vi "PPMS_CREA_SECUENCIA.vi"(8 "error in (no error)":errorcluster) -> (0 "error out":errorcluster, 1 "Total":string[](array[string]), 2 "Pasos":i32, 3 "Secuencia":string[](array[string]))   [LabVIEW 2017]
uses:
  <vilib>/Utility/file.llb/Read Delimited Spreadsheet (string).vi
panel:
  out "idxScanVi":i16
  out "idxScanVf":i16
  out "Scan V":bool
  out "subArray2D":string[][](array[string])
  out "Seq scans":string[](array[string])
  out "Seq final":string[](array[string])
  out "Seq inicial":string[](array[string])
  out "idxScanTi":i16
  out "idxScanFi":i16
  out "idxScanFf":i16
  out "idxScanTf":i16
  out "Array2D":string[][](array[string])
  out "Scan T":bool
  out "Scan F":bool
  in  "Salir":bool
  in  "Borra linea":bool
  in  "Grabar":bool
  in  "Cargar":bool
  out "SequenceFile":path
  in  "Command line (double click)":i32(listbox) caption="Válvulas"
  in  "Secuencia":i32(listbox)=-1
  # "Septiembre 2019 V1.2  a-sslcdms"
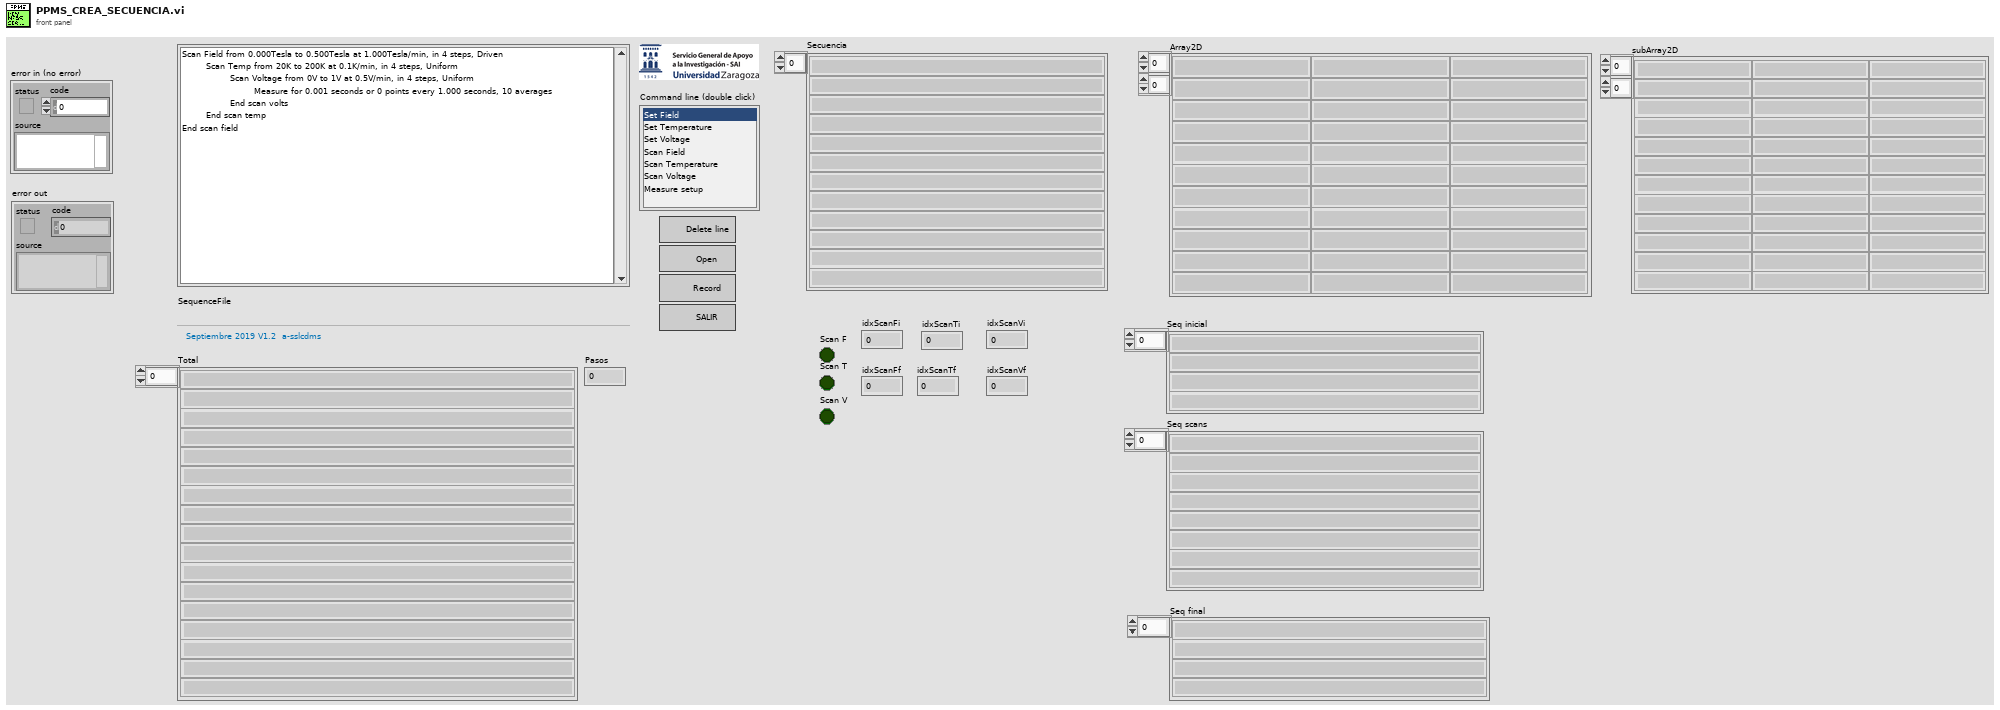
[diagram p1: front panel]
types:
  T1 = enum16{"open", "open or create", "create or replace", "create", "open (read only)"}
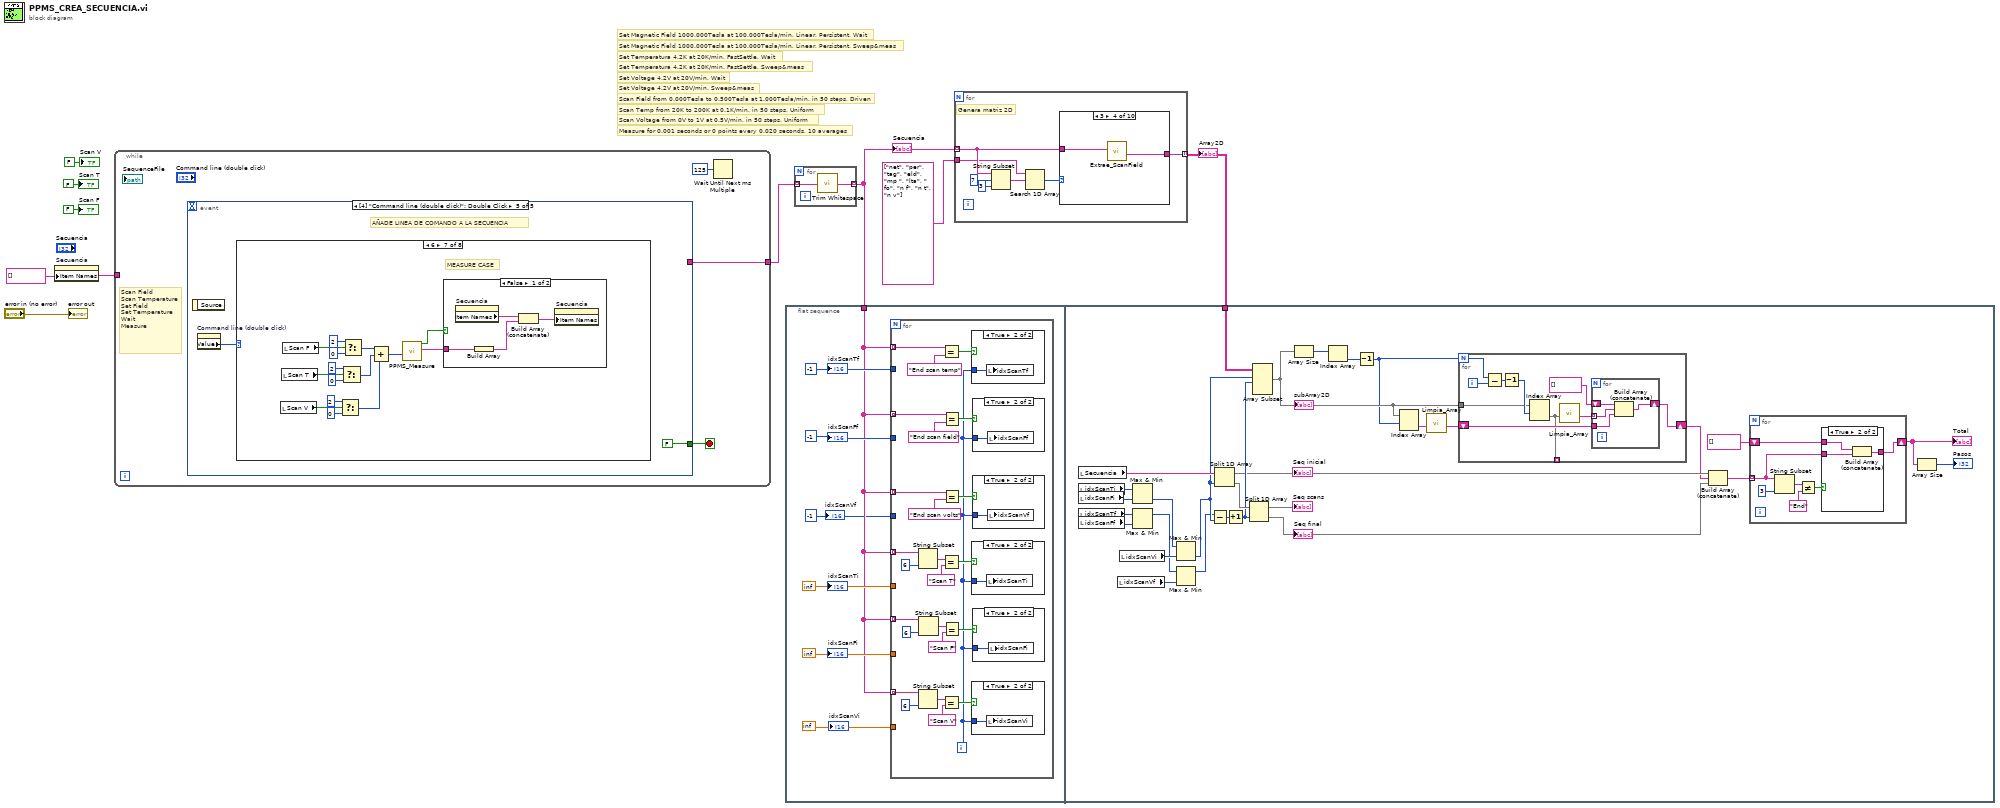
[diagram p0: block diagram]
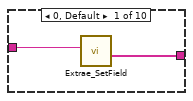
[diagram p9: hidden frame]
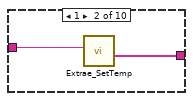
[diagram p10: hidden frame]
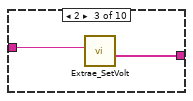
[diagram p11: hidden frame]
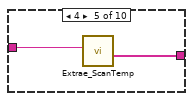
[diagram p12: hidden frame]
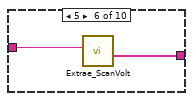
[diagram p13: hidden frame]
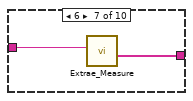
[diagram p14: hidden frame]
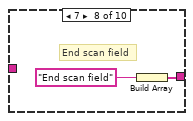
[diagram p15: hidden frame]
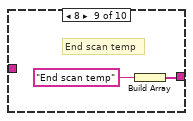
[diagram p16: hidden frame]
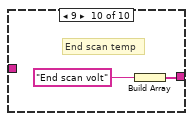
[diagram p17: hidden frame]
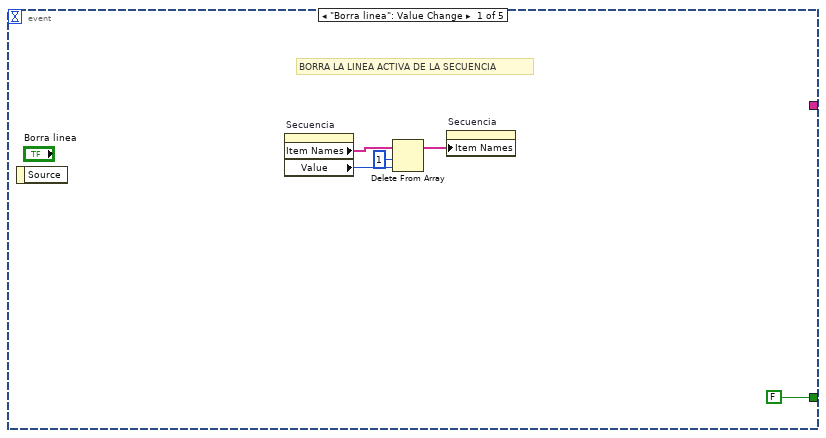
[diagram p18: hidden frame]
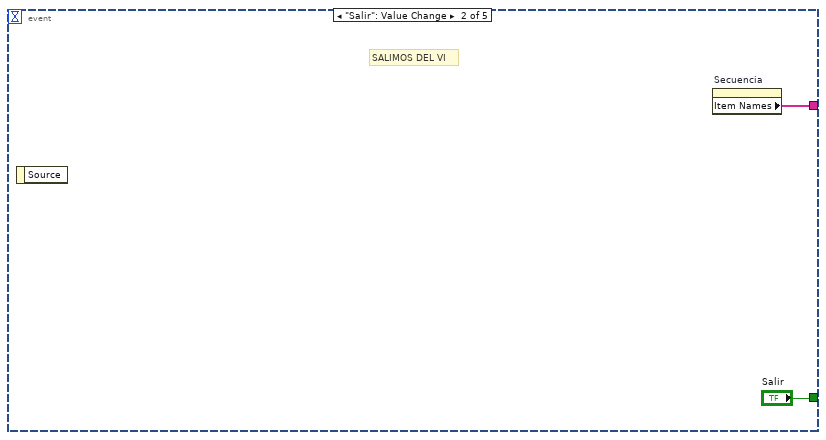
[diagram p19: hidden frame]
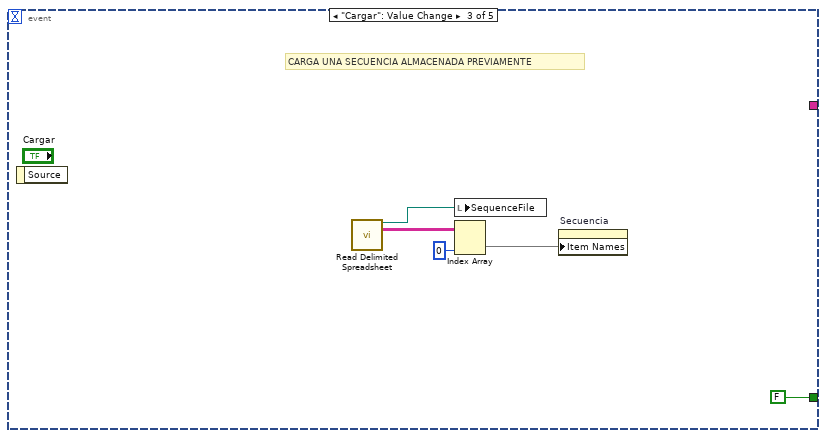
[diagram p20: hidden frame]
diagram:
  w9 = string[] [] ("Item Names")
  # "Measure for 0.001 seconds or 0 points every 0.020 seconds, 10 averages"
  # "Scan Voltage from 0V to 1V at 0.5V/min, in 50 steps, Uniform"
  # "Scan Temp from 20K to 200K at 0.1K/min, in 50 steps, Uniform"
  # "Scan Field from 0.000Tesla to 0.500Tesla at 1.000Tesla/min, in 50 steps, Driven"
  # "Set Temperatura 4.2K at 20K/min, FastSettle, Sweep&meas"
  # "Set Temperatura 4.2K at 20K/min, FastSettle, Wait"
  # "Set Magnetic Field 1000.000Tesla at 100.000Tesla/min, Linear, Persistent, Sweep&meas"
  # "Set Magnetic Field 1000.000Tesla at 100.000Tesla/min, Linear, Persistent, Wait"
  # "Set Voltage 4.2V at 20V/min, Sweep&meas"
  # "Set Voltage 4.2V at 20V/min, Wait"
  n1 = property on="Secuencia" class="LstBox (strict)"("Item Names"=w9) -> ()  [unwired: 2 in, 2 out]
  n2 = while {
    tunnel: w9 -> [_]
    tunnel: [w10] -> w4
    stop <- w11 stop-if-true
    # "Scan Field\nScan Temperature\nSet Field\nSet Temperature\nWait\nMeasure"
    n3 = event shown="[4] \"Command line (double click)\": Double Click" {
      selector: _ -> [_ _ _ _ _]
      dyn-events: _ -> [_ _ _ _ _]
      timeout: _ -> [_ _ _ _ _]
      tunnel: [FALSE ("Salir") "Salir" FALSE ("Salir") FALSE ("Salir") FALSE ("Salir")] -> w11
      tunnel: [_ w18 _ _ _] -> w10
      event "Borra linea": Value Change {
        # "BORRA LA LINEA ACTIVA DE LA SECUENCIA"
        n4 = event-data() -> ()  [unwired: 1 in, 1 out]
        n5 = property on="Secuencia" class="LstBox (strict)"() -> ("Item Names"=w17:string[], "Value"=w16:i32)  [unwired: 2 in, 2 out]
        n6 = Delete From Array(array=w17, length=1, index=w16) -> (array with subset deleted=w14:string[])  [unwired: 1 out]
        n7 = property on="Secuencia" class="LstBox (strict)"("Item Names"=w14) -> ()  [unwired: 2 in, 2 out]
      }
      event "Salir": Value Change {
        # "SALIMOS DEL VI"
        n8 = event-data() -> ()  [unwired: 1 in, 1 out]
        n9 = property on="Secuencia" class="LstBox (strict)"() -> ("Item Names"=w18:string[])  [unwired: 2 in, 2 out]
      }
      event "Cargar": Value Change {
        # "CARGA UNA SECUENCIA ALMACENADA PREVIAMENTE"
        n10 = event-data() -> ()  [unwired: 1 in, 1 out]
        n11 = call-poly <vilib>:"Read Delimited Spreadsheet.vi"() -> ("new file path (Not A Path if cancelled)"=w21:path, "all rows"=w20:string[][])  [unwired: 10 in, 4 out]
        n12 = local write "SequenceFile"(w21) -> ()
        n13 = Index Array(array=w20, index (col)=0 ("disabled index (col)")) -> (element=w22:string[])  [unwired: 1 in]
        n14 = property on="Secuencia" class="LstBox (strict)"("Item Names"=w22) -> ()  [unwired: 2 in, 2 out]
      }
      event "Grabar": Value Change {
        # "GRABA UNA SECUENCIA PARA USAR MAS ADELANTE"
        n15 = event-data() -> ()  [unwired: 1 in, 1 out]
        n16 = property on="Secuencia" class="LstBox (strict)"() -> ("Item Names"=w28:string[])  [unwired: 2 in, 2 out]
        n17 = call <vilib>:"Open_Create_Replace File.vi"("function (open:0)"=T1."create or replace") -> ("new file path"=w25:path)  [unwired: 7 in, 3 out]
        n18 = local write "SequenceFile"(w25) -> ()
        n19 = for {
          tunnel: w28 -> [w31] mode=indexing
          shift-right: [w33] -> _
          shift-left: w25 -> [w34]
          n20 = Concatenate Strings(w31, "\r\n") -> (w30:string)
          n21 = call <vilib>:"Write Characters To File.vi"("append to file? (new file:F)"=TRUE, "character string"=w30, "file path (dialog if empty)"=w34) -> ("new file path (Not A Path if cancelled)"=w33:path)  [unwired: 2 in]
        }
      }
      event "Command line (double click)": Double Click {
        # "AÑADE LINEA DE COMANDO A LA SECUENCIA"
        n22 = event-data() -> ()  [unwired: 1 in, 1 out]
        n23 = property on="Command line (double click)" class="LstBox (strict)"() -> ("Value"=w35:i32)  [unwired: 2 in, 2 out]
        n24 = case shown="6" w35 {
          frame 0, Default {
            # "SET FIELD"
            n25 = call "PPMS_SetCampo.vi"("Index"=i8 0) -> ("resulting string 1"=w38:string, "Cancelled?"=w39:bool)  [unwired: 6 in, 1 out]
            n26 = case shown="False" w39 {
              tunnel: w38 -> [w40 _]
              frame False {
                n27 = property on="Secuencia" class="LstBox (strict)"() -> ("Item Names"=w41:string[])  [unwired: 2 in, 2 out]
                n28 = Build Array (concatenate)(w41, w40) -> (w42:string[])
                n29 = property on="Secuencia" class="LstBox (strict)"("Item Names"=w42) -> ()  [unwired: 2 in, 2 out]
              }
              frame True {
              }
            }
          }
          frame 1 {
            # "SET TEMPERATURE"
            n30 = call "PPMS_SetTemperatura.vi"("Index"=i8 0) -> ("resulting string 1"=w44:string, "Cancelled?"=w45:bool)  [unwired: 6 in, 1 out]
            n31 = case shown="False" w45 {
              tunnel: w44 -> [w46 _]
              frame False {
                n32 = property on="Secuencia" class="LstBox (strict)"() -> ("Item Names"=w48:string[])  [unwired: 2 in, 2 out]
                n33 = Build Array (concatenate)(w48, w46) -> (w47:string[])
                n34 = property on="Secuencia" class="LstBox (strict)"("Item Names"=w47) -> ()  [unwired: 2 in, 2 out]
              }
              frame True {
              }
            }
          }
          frame 2 {
            # "SET VOLTAGE"
            n35 = call "PPMS_SetVoltage.vi"("Index"=i8 0) -> ("resulting string 1"=w49:string, "Cancelled?"=w50:bool)  [unwired: 6 in, 1 out]
            n36 = case shown="False" w50 {
              tunnel: w49 -> [w54 _]
              frame False {
                n37 = property on="Secuencia" class="LstBox (strict)"() -> ("Item Names"=w53:string[])  [unwired: 2 in, 2 out]
                n38 = Build Array (concatenate)(w53, w54) -> (w52:string[])
                n39 = property on="Secuencia" class="LstBox (strict)"("Item Names"=w52) -> ()  [unwired: 2 in, 2 out]
              }
              frame True {
              }
            }
          }
          frame 3 {
            # "SCAN FIELD"
            n40 = local read "Scan F"() -> (w55:bool)
            n41 = case shown="False" w55 {
              frame False {
                n42 = local read "Scan T"() -> (w61:bool)
                n43 = local read "Scan V"() -> (w62:bool)
                n44 = Select(t=i8 2 ("Index"), s=w61, f=i8 0 ("Index")) -> (s? t:f=w57:i8)
                n45 = Select(t=i8 2 ("Index"), s=w62, f=i8 0 ("Index")) -> (s? t:f=w58:i8)
                n46 = Add(x=w58, y=w57) -> (x+y=w56:i8)
                n47 = local write "Scan F"(TRUE ("Scan T")) -> ()
                n48 = call "PPMS_ScanCampo.vi"("Index"=w56) -> ("resulting string 2"=w67:string, "resulting string 1"=w68:string, "Cancelled?"=w66:bool)  [unwired: 5 in, 1 out]
                n49 = case shown="False" w66 {
                  tunnel: w68 -> [w73 _]
                  tunnel: w67 -> [w72 _]
                  frame False {
                    n50 = property on="Secuencia" class="LstBox (strict)"() -> ("Item Names"=w71:string[])  [unwired: 2 in, 2 out]
                    n51 = Build Array(w73, w72) -> (w70:string[])
                    n52 = Build Array (concatenate)(w71, w70) -> (w69:string[])
                    n53 = property on="Secuencia" class="LstBox (strict)"("Item Names"=w69) -> ()  [unwired: 2 in, 2 out]
                  }
                  frame True {
                  }
                }
              }
              frame True {
                n54 = One Button Dialog(message="Solo esta permitido\nun scan de campo por secuencia") -> ()  [unwired: 1 in, 1 out]
              }
            }
          }
          frame 4 {
            # "SCAN TEMPERATURE"
            n55 = local read "Scan T"() -> (w75:bool)
            n56 = case shown="False" w75 {
              frame False {
                n57 = local read "Scan V"() -> (w81:bool)
                n58 = local read "Scan F"() -> (w82:bool)
                n59 = local write "Scan T"(TRUE ("Scan T")) -> ()
                n60 = Select(t=i8 2 ("Index"), s=w81, f=i8 0 ("Index")) -> (s? t:f=w77:i8)
                n61 = Select(t=i8 2 ("Index"), s=w82, f=i8 0 ("Index")) -> (s? t:f=w78:i8)
                n62 = Add(x=w78, y=w77) -> (x+y=w76:i8)
                n63 = call "PPMS_ScanTemperatura.vi"("Index"=w76) -> ("resulting string 2"=w86:string, "resulting string 1"=w87:string, "Cancelled?"=w88:bool)  [unwired: 5 in, 1 out]
                n64 = case shown="False" w88 {
                  tunnel: w87 -> [w93 _]
                  tunnel: w86 -> [w92 _]
                  frame False {
                    n65 = property on="Secuencia" class="LstBox (strict)"() -> ("Item Names"=w91:string[])  [unwired: 2 in, 2 out]
                    n66 = Build Array(w93, w92) -> (w90:string[])
                    n67 = Build Array (concatenate)(w91, w90) -> (w89:string[])
                    n68 = property on="Secuencia" class="LstBox (strict)"("Item Names"=w89) -> ()  [unwired: 2 in, 2 out]
                  }
                  frame True {
                  }
                }
              }
              frame True {
                n69 = One Button Dialog(message="Solo esta permitido\nun scan de temperatura por secuencia") -> ()  [unwired: 1 in, 1 out]
              }
            }
          }
          frame 5 {
            # "SCAN VOLTAGE"
            n70 = local read "Scan V"() -> (w95:bool)
            n71 = case shown="False" w95 {
              frame False {
                n72 = local read "Scan T"() -> (w103:bool)
                n73 = local read "Scan F"() -> (w104:bool)
                n74 = local write "Scan V"(TRUE ("Scan T")) -> ()
                n75 = Select(t=i8 2 ("Index"), s=w103, f=i8 0 ("Index")) -> (s? t:f=w101:i8)
                n76 = Select(t=i8 2 ("Index"), s=w104, f=i8 0 ("Index")) -> (s? t:f=w102:i8)
                n77 = Add(x=w102, y=w101) -> (x+y=w96:i8)
                n78 = call "PPMS_ScanVoltage.vi"("Index"=w96) -> ("resulting string 2"=w106:string, "resulting string 1"=w107:string, "Cancelled?"=w108:bool)  [unwired: 5 in, 1 out]
                n79 = case shown="False" w108 {
                  tunnel: w107 -> [w113 _]
                  tunnel: w106 -> [w112 _]
                  frame False {
                    n80 = property on="Secuencia" class="LstBox (strict)"() -> ("Item Names"=w111:string[])  [unwired: 2 in, 2 out]
                    n81 = Build Array(w113, w112) -> (w110:string[])
                    n82 = Build Array (concatenate)(w111, w110) -> (w109:string[])
                    n83 = property on="Secuencia" class="LstBox (strict)"("Item Names"=w109) -> ()  [unwired: 2 in, 2 out]
                  }
                  frame True {
                  }
                }
              }
              frame True {
                n84 = One Button Dialog(message="Solo esta permitido\nun scan de temperatura por secuencia") -> ()  [unwired: 1 in, 1 out]
              }
            }
          }
          frame 6 {
            # "MEASURE CASE"
            n85 = local read "Scan V"() -> (w116:bool)
            n86 = local read "Scan T"() -> (w124:bool)
            n87 = local read "Scan F"() -> (w125:bool)
            n88 = Select(t=i8 2 ("Index"), s=w116, f=i8 0 ("Index")) -> (s? t:f=w115:i8)
            n89 = Select(t=i8 2 ("Index"), s=w124, f=i8 0 ("Index")) -> (s? t:f=w120:i8)
            n90 = Select(t=i8 2 ("Index"), s=w125, f=i8 0 ("Index")) -> (s? t:f=w121:i8)
            n91 = Compound Arithmetic op=ADD(w121, w120, w115) -> (w119:i8)
            n92 = call "PPMS_Measure.vi"("Index"=w119) -> ("resulting string 1"=w128:string, "Cancelled?"=w129:bool)  [unwired: 6 in, 1 out]
            n93 = case shown="False" w129 {
              tunnel: w128 -> [w133 _]
              frame False {
                n94 = property on="Secuencia" class="LstBox (strict)"() -> ("Item Names"=w131:string[])  [unwired: 2 in, 2 out]
                n95 = Build Array(w133) -> (w130:string[])
                n96 = Build Array (concatenate)(w131, w130) -> (w132:string[])
                n97 = property on="Secuencia" class="LstBox (strict)"("Item Names"=w132) -> ()  [unwired: 2 in, 2 out]
              }
              frame True {
              }
            }
          }
          frame 7 {
            # "End Program"
            n98 = property on="Secuencia" class="LstBox (strict)"() -> ("Item Names"=w134:string[])  [unwired: 2 in, 2 out]
            n99 = Build Array (concatenate)(w134, "End Program" ("message")) -> ()  [unwired: 1 out]
            n100 = property on="Secuencia" class="LstBox (strict)"("Item Names"=w134) -> ()  [unwired: 2 in, 2 out]
          }
        }
      }
    }
    n101 = Wait Until Next ms Multiple(millisecond multiple=u32 125) -> ()  [unwired: 1 out]
  }
  n102 = flat-sequence {
    tunnel: w3 -> [w138]
    tunnel: w2 -> [w194]
    frame #0 {
      w137 = i16 -1 ("idxScanT")
      w136 = inf
      w139 = inf
      w140 = inf
      w141 = i16 -1 ("idxScanT")
      w142 = i16 -1 ("idxScanT")
      n103 = for {
        tunnel: w138 -> [w158] mode=indexing
        tunnel: w142 -> [_]
        tunnel: w138 -> [w157] mode=indexing
        tunnel: w141 -> [_]
        tunnel: w138 -> [w155] mode=indexing
        tunnel: w138 -> [w154] mode=indexing
        tunnel: w139 -> [_]
        tunnel: w140 -> [_]
        tunnel: w138 -> [w150] mode=indexing
        tunnel: w136 -> [_]
        tunnel: w138 -> [w146] mode=indexing
        tunnel: w137 -> [_]
        i -> [w143]
        n104 = String Subset(string=w155, length (rest)=6 ("length (rest)")) -> (substring=w152:string)  [unwired: 1 in]
        n105 = String Subset(string=w150, length (rest)=6 ("length (rest)")) -> (substring=w151:string)  [unwired: 1 in]
        n106 = String Subset(string=w154, length (rest)=6 ("length (rest)")) -> (substring=w153:string)  [unwired: 1 in]
        n107 = Equal?(x=w158, y="End scan temp" ("trimmed string")) -> (x = y?=w166:bool)
        n108 = Equal?(x=w152, y="Scan T" ("trimmed string")) -> (x = y?=w161:bool)
        n109 = Equal?(x=w151, y="Scan V" ("trimmed string")) -> (x = y?=w148:bool)
        n110 = Equal?(x=w157, y="End scan field" ("trimmed string")) -> (x = y?=w165:bool)
        n111 = Equal?(x=w146, y="End scan volts" ("trimmed string")) -> (x = y?=w144:bool)
        n112 = Equal?(x=w153, y="Scan F" ("trimmed string")) -> (x = y?=w162:bool)
        n113 = case shown="True" w166 {
          tunnel: w143 -> [_ w173]
          frame False {
          }
          frame True {
            n114 = local write "idxScanTf"(w173) -> ()
          }
        }
        n115 = case shown="True" w161 {
          tunnel: w143 -> [_ w171]
          frame False {
          }
          frame True {
            n116 = local write "idxScanTi"(w171) -> ()
          }
        }
        n117 = case shown="True" w148 {
          tunnel: w143 -> [_ w169]
          frame False {
          }
          frame True {
            n118 = local write "idxScanVi"(w169) -> ()
          }
        }
        n119 = case shown="True" w165 {
          tunnel: w143 -> [_ w172]
          frame False {
          }
          frame True {
            n120 = local write "idxScanFf"(w172) -> ()
          }
        }
        n121 = case shown="True" w144 {
          tunnel: w143 -> [_ w168]
          frame False {
          }
          frame True {
            n122 = local write "idxScanVf"(w168) -> ()
          }
        }
        n123 = case shown="True" w162 {
          tunnel: w143 -> [_ w170]
          frame False {
          }
          frame True {
            n124 = local write "idxScanFi"(w170) -> ()
          }
        }
      }
      "idxScanTf" <- w142
      "idxScanFf" <- w141
      "idxScanTi" <- w140
      "idxScanFi" <- w139
      "idxScanVf" <- w137
      "idxScanVi" <- w136
    }
    frame #1 {
      n125 = local read "Secuencia"() -> (w202:string[])
      n126 = local read "idxScanTi"() -> (w201:i16)
      n127 = local read "idxScanFi"() -> (w200:i16)
      n128 = local read "idxScanTf"() -> (w198:i16)
      n129 = local read "idxScanFf"() -> (w199:i16)
      n130 = local read "idxScanVf"() -> (w179:i16)
      n131 = local read "idxScanVi"() -> (w178:i16)
      n132 = Max & Min(x=w201, y=w200) -> (min(x,y)=w177:i16)  [unwired: 1 out]
      n133 = Max & Min(x=w198, y=w199) -> (max(x,y)=w175:i16)  [unwired: 1 out]
      n134 = Max & Min(x=w177, y=w178) -> (min(x,y)=w176:i16)  [unwired: 1 out]
      n135 = Max & Min(x=w175, y=w179) -> (max(x,y)=w174:i16)  [unwired: 1 out]
      n136 = Subtract(x=w174, y=w176) -> (x-y=w195:i16)
      n137 = Split 1D Array(array=w202, index=w176) -> (first subarray=w185:string[], second subarray=w196:string[])
      "Seq inicial" <- w185
      n138 = Increment(x=w195) -> (x+1=w193:i16)
      n139 = Split 1D Array(array=w196, index=w193) -> (first subarray=→"Seq scans":string[], second subarray=w186:string[])
      "Seq final" <- w186
      n140 = Array Subset(array=w194, index (row)=w176, length (row)=w193) -> (w190:string[][])  [unwired: 2 in]
      "subArray2D" <- w190
      n141 = Array Size(array=w190) -> (size(s)=w189:i32[])
      n142 = Index Array(array=w189) -> (element=w188:i32)  [unwired: 1 in]
      n143 = Decrement(x=w188) -> (x-1=w187:i32)
      n144 = Index Array(array=w190, index (row)=w187) -> (element=w191:string[])  [unwired: 1 in]
      n145 = call "Limpia_Array.vi"("Array in"=w191) -> ("Array out"=w192:string[])  [unwired: 10 in]
      n146 = for {
        N: w187 -> [w223]
        tunnel: w190 -> [w220]
        shift-right: [w216] -> w184
        shift-left: w192 -> [w217]
        tunnel: [w214] -> _ mode=indexing
        i -> [w222]
        n147 = Subtract(x=w223, y=w222) -> (x-y=w219:i32)
        n148 = Decrement(x=w219) -> (x-1=w221:i32)
        n149 = Index Array(array=w220, index (row)=w221) -> (element=w214:string[])  [unwired: 1 in]
        n150 = call "Limpia_Array.vi"("Array in"=w214) -> ("Array out"=w215:string[])  [unwired: 10 in]
        n151 = for {
          tunnel: w215 -> [w226] mode=indexing
          shift-right: [w224] -> w216
          shift-left: string[] [] -> [w227]
          tunnel: w217 -> [w225]
          n152 = Build Array (concatenate)(w227, w226, w225) -> (w224:string[])
        }
      }
      n153 = Build Array (concatenate)(w185, w184, w186) -> (w183:string[])
      n154 = for {
        tunnel: w183 -> [w203] mode=indexing
        shift-right: [w205] -> w181
        shift-left: string[] [] -> [w206]
        n155 = String Subset(string=w203, length (rest)=3 ("length (rest)")) -> (substring=w209:string)  [unwired: 1 in]
        n156 = Not Equal?(x=w209, y="End" ("trimmed string")) -> (x != y?=w204:bool)
        n157 = case shown="True" w204 {
          tunnel: w206 -> [w210 w213]
          tunnel: [w210 w212] -> w205
          tunnel: w203 -> [_ w211]
          frame False {
          }
          frame True {
            n158 = Build Array (concatenate)(w213, w211) -> (w212:string[])
          }
        }
      }
      "Total" <- w181
      n159 = Array Size(array=w181) -> (size(s)=→"Pasos":i32)
    }
  }
  n160 = for {
    tunnel: w4 -> [w229] mode=indexing
    tunnel: [w228] -> w3 mode=indexing
    n161 = call <vilib>:"Trim Whitespace.vi"("string"=w229) -> ("trimmed string"=w228:string)  [unwired: 1 in]
  }
  "Secuencia" <- w3
  n162 = for {
    tunnel: w3 -> [w231] mode=indexing
    tunnel: [w232] -> w2 mode=indexing
    tunnel: string[] ["net", "per", "tag", "eld", "mp ", "lta", " fo", "n f", "n t", "n v"] ("Array") -> [w230]
    # "Genera matriz 2D"
    n163 = String Subset(string=w231, offset (0)=7, length (rest)=3 ("length (rest)")) -> (substring=w234:string)
    n164 = Search 1D Array(1D array=w230, element=w234) -> (index of element=w233:i32)  [unwired: 1 in]
    n165 = case shown="3" w233 {
      tunnel: w231 -> [w238 w240 w242 w244 w246 w248 w250 _ _ _]
      tunnel: [w237 w239 w241 w243 w245 w247 w249 w251 w253 w255] -> w232
      frame 0, Default {
        n166 = call "Extrae_SetField.vi"("String"=w238) -> ("Array"=w237:string[])  [unwired: 10 in]
      }
      frame 1 {
        n167 = call "Extrae_SetTemp.vi"("String"=w240) -> ("Array"=w239:string[])  [unwired: 10 in]
      }
      frame 2 {
        n168 = call "Extrae_SetVolt.vi"("String"=w242) -> ("Array"=w241:string[])  [unwired: 10 in]
      }
      frame 3 {
        n169 = call "Extrae_ScanField.vi"("F string"=w244) -> ("Array F"=w243:string[])  [unwired: 10 in]
      }
      frame 4 {
        n170 = call "Extrae_ScanTemp.vi"("T string"=w246) -> ("Array T"=w245:string[])  [unwired: 10 in]
      }
      frame 5 {
        n171 = call "Extrae_ScanVolt.vi"("V string"=w248) -> ("Array V"=w247:string[])  [unwired: 10 in]
      }
      frame 6 {
        n172 = call "Extrae_Measure.vi"("String"=w250) -> ("Array"=w249:string[])  [unwired: 10 in]
      }
      frame 7 {
        # "End scan field"
        n173 = Build Array("End scan field" ("trimmed string")) -> (w251:string[])
      }
      frame 8 {
        # "End scan temp"
        n174 = Build Array("End scan temp" ("trimmed string")) -> (w253:string[])
      }
      frame 9 {
        # "End scan temp"
        n175 = Build Array("End scan volt" ("trimmed string")) -> (w255:string[])
      }
    }
  }
  "Array2D" <- w2
  "error out" <- "error in (no error)"
  "Scan F" <- FALSE ("Loop H")
  "Scan T" <- FALSE ("Loop T")
  "Scan V" <- FALSE ("Loop T")
